vi "Remove DC.vi"(1 "FFT in":cdb[](array[numeric])) -> (0 "FFT out":cdb[](array[numeric]))   [LabVIEW 2021, in "RTL-SDR.lvlib"]
uses:
  RTL-SDR.lvlib
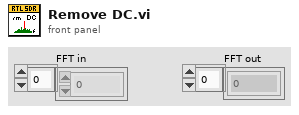
[diagram p1: front panel]
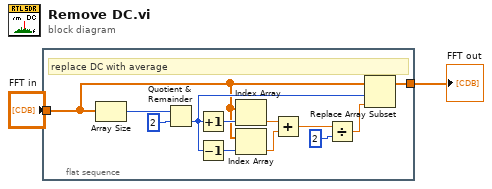
[diagram p0: block diagram]
diagram:
  n1 = flat-sequence {
    tunnel: "FFT in" -> [w7]
    tunnel: [w3] -> w2
    frame #0 {
      # "replace DC with average"
      n2 = Array Size(array=w7) -> (size(s)=w14:i32)
      n3 = Quotient & Remainder(x=w14, y=2) -> (floor(x/y)=w10:i32)  [unwired: 1 out]
      n4 = Increment(x=w10) -> (x+1=w11:i32)
      n5 = Decrement(x=w10) -> (x-1=w12:i32)
      n6 = Index Array(array=w7, index=w11) -> (element=w9:cdb)
      n7 = Index Array(array=w7, index=w12) -> (element=w8:cdb)
      n8 = Add(x=w9, y=w8) -> (x+y=w6:cdb)
      n9 = Divide(x=w6, y=2) -> (x/y=w4:cdb)
      n10 = Replace Array Subset(array=w7, new element=w4, index=w10) -> (w3:cdb[])
    }
  }
  "FFT out" <- w2
